vi "Read String.vi"(11 "GDSII.DataType.String in":refnum<class "GDSII.DataType.String.lvclass">) -> (2 "String":string, 3 "GDSII.DataType.String out":refnum<class "GDSII.DataType.String.lvclass">)   [LabVIEW 2019, in "GDSII.DataType.String.lvclass"]
uses:
  GDSII.DataType.String.lvclass
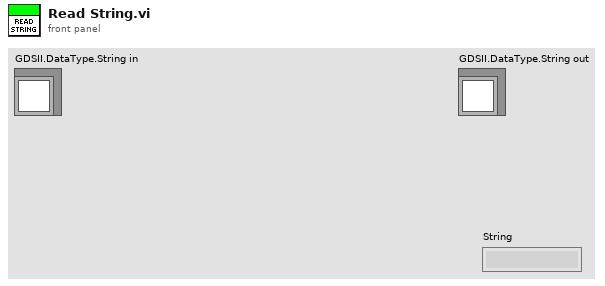
[diagram p1: front panel]
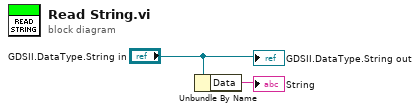
[diagram p0: block diagram]
diagram:
  n1 = Unbundle By Name("GDSII.DataType.String in") -> ("Data"=→"String":string)
  "GDSII.DataType.String out" <- "GDSII.DataType.String in"
